vi "SpecAn Ref Level Set.vi"(0 "VISA In":refnum<visa-resource-name>, 5 "Error In":errorcluster, 6 "Amplitude Units (0: dBm)":i32(ring) items=["dBm", "dBmV", "dBmA", "W", "V", "A", "dBuV", "dBuA"], 8 "Reference Level Offset (0 dB)":dbl, 10 "Reference Level (0 dBm)":dbl) -> (14 "VISA Out":refnum<visa-resource-name>, 19 "Error Out":errorcluster)   [LabVIEW 2015]
uses:
  Controls/FGV Action SpecAn Model.ctl
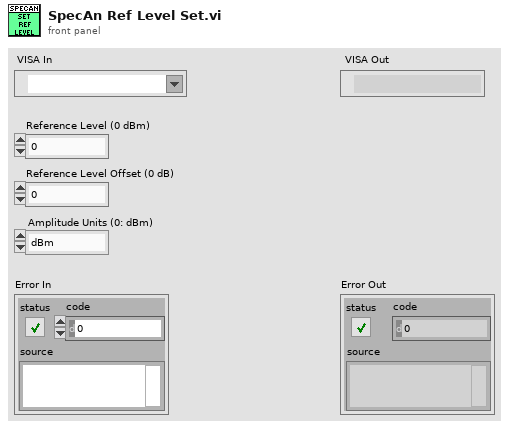
[diagram p1: front panel]
types:
  T1 = typedef "FGV Action SpecAn Model.ctl" = enum16{"Get", "Set"}
  T2 = typedef "SpecAn Model.ctl" = enum16{"E4440", "N9030"}
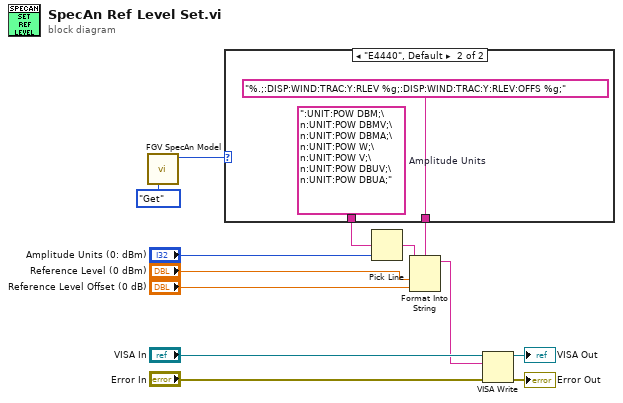
[diagram p0: block diagram]
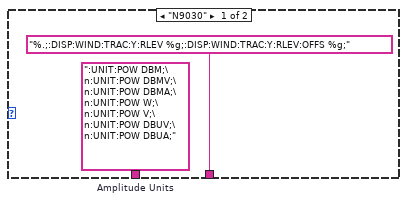
[diagram p2: hidden frame]
diagram:
  n1 = call "FGV SpecAn Model.vi"("Action"=FGV_Action_SpecAn_Model."Get") -> ("SA Model"=w1:T2)  [unwired: 6 in, 1 out]
  n2 = case shown="\"E4440\", Default" w1 {
    tunnel: ["%.;:DISP:WIND:TRAC:Y:RLEV %g;:DISP:WIND:TRAC:Y:RLEV:OFFS %g;" ("format string") "%.;:DISP:WIND:TRAC:Y:RLEV %g;:DISP:WIND:TRAC:Y:RLEV:OFFS %g;" ("format string")] -> w6
    tunnel: [w14 w16] -> w4
    frame "N9030" {
      w14 = ":UNIT:POW DBM;\n:UNIT:POW DBMV;\n:UNIT:POW DBMA;\n:UNIT:POW W;\n:UNIT:POW V;\n:UNIT:POW DBUV;\n:UNIT:POW DBUA;"  # Amplitude Units
    }
    frame "E4440", Default {
      w16 = ":UNIT:POW DBM;\n:UNIT:POW DBMV;\n:UNIT:POW DBMA;\n:UNIT:POW W;\n:UNIT:POW V;\n:UNIT:POW DBUV;\n:UNIT:POW DBUA;"  # Amplitude Units
    }
  }
  n3 = Pick Line(multi-line string=w4, line index="Amplitude Units (0: dBm)") -> (output string=w5:string)  [unwired: 1 in]
  n4 = Format Into String(format string=w6, initial string=w5, "Reference Level (0 dBm)", "Reference Level Offset (0 dB)") -> (resulting string=w3:string)  [unwired: 1 in, 1 out]
  n5 = VISA Write(VISA resource name="VISA In", write buffer=w3, error in (no error)="Error In") -> (VISA resource name out=→"VISA Out":refnum<visa-resource-name>, error out=→"Error Out":errorcluster)  [unwired: 1 out]
